vi "Get Connections.vi"(6 "instrument type id":string, 7 "error if pin not found":bool, 8 "error in":errorcluster, 9 "sites":i32[](array[numeric]), 10 "pin or relay names":string[](array[string]), 11 "connection map in":refnum<class "Connection Map.lvclass">) -> (0 "error out":errorcluster, 2 "connections":T1[](array[typedef]), 3 "connection map out":refnum<class "Connection Map.lvclass">)   [LabVIEW 2020, in "MeasurementLink Session Management.lvlib" / "Connection Map.lvclass"]
uses:
  Connection Map.lvclass
  Session Reservation/Connection with Session.ctl
  Session Reservation/Connection.ctl
  Connection Map.lvclass/Connection Map.ctl
  41d5ce38-2fc1-4a99-b6dc-ff10a635fcc4.vi
  MeasurementLink Measurement Server/Helpers/Error Strings Global Internal.vi
  Session Reservation/Session Reservation.lvclass
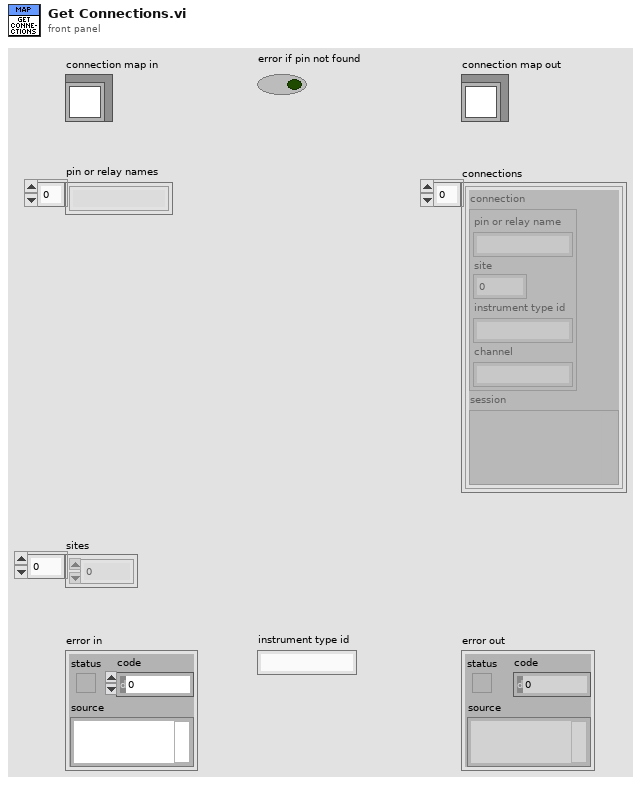
[diagram p1: front panel]
types:
  T1 = typedef "MeasurementLink Session Management.lvlib/Session Reservation.lvclass/Connection with Session.ctl" = cluster{"connection":T2, "session":variant}
  T2 = typedef "MeasurementLink Session Management.lvlib/Session Reservation.lvclass/Connection.ctl" = cluster{"pin or relay name":string, "site":i32, "instrument type id":string, "channel":string}
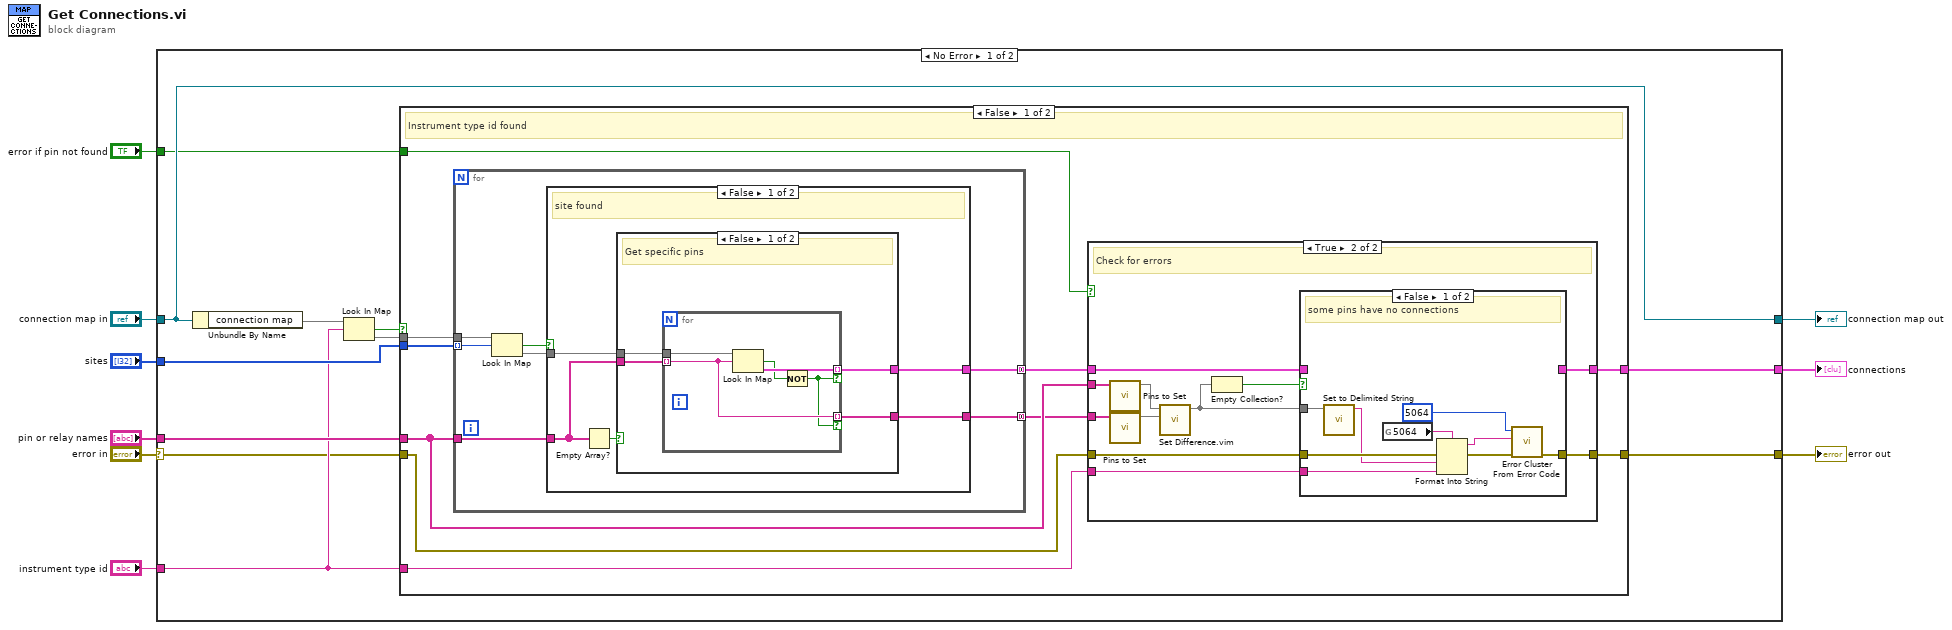
[diagram p0: block diagram]
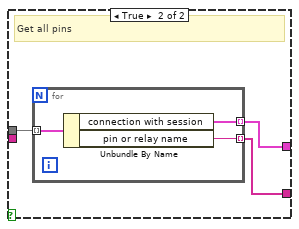
[diagram p2: hidden frame]
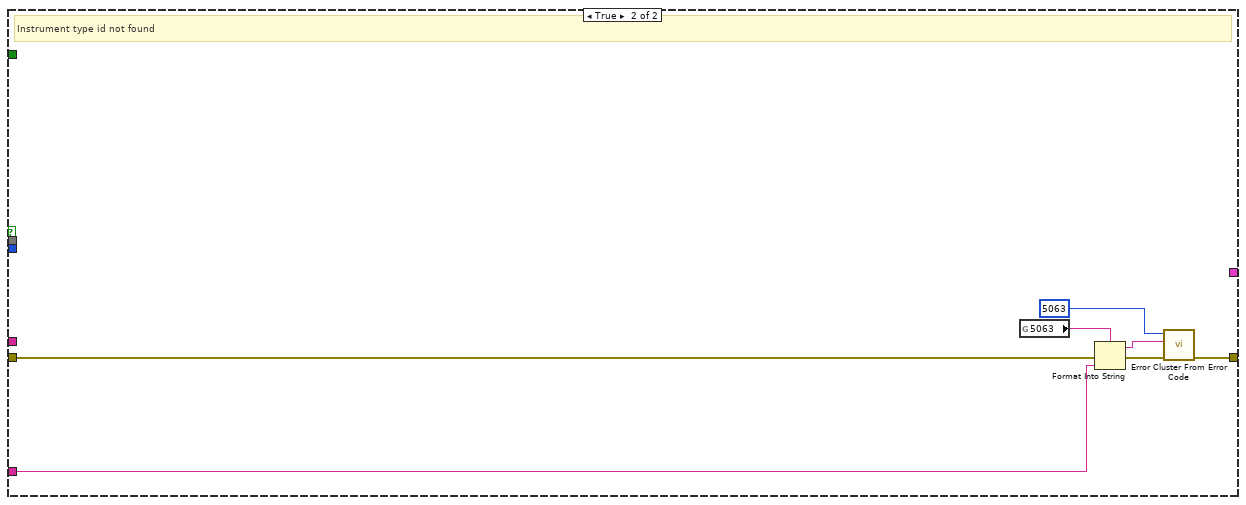
[diagram p6: hidden frame]
diagram:
  n1 = case shown="No Error" "error in" {
    selector: "error in" -> [w11 w90]
    tunnel: [w14 w90] -> w8
    tunnel: [w16 w89] -> w6
    tunnel: "connection map in" -> [w16 w89]
    tunnel: "instrument type id" -> [w13 _]
    tunnel: "sites" -> [w18 _]
    tunnel: "pin or relay names" -> [w17 _]
    tunnel: [w10 _] -> w2
    tunnel: "error if pin not found" -> [w12 _]
    frame No Error {
      n2 = Unbundle By Name(w16) -> ("connection map"=w15:map{string, map{i32, map{string, T1}}})
      n3 = Look In Map(map=w15, key=w13) -> (key not found?=w19:bool, value=w20:map{i32, map{string, T1}})  [unwired: 1 in]
      n4 = case shown="False" w19 {
        tunnel: w20 -> [w30 _]
        tunnel: w18 -> [w29 _]
        tunnel: w17 -> [w22 _]
        tunnel: [w28 _] -> w10
        tunnel: w11 -> [w24 w88]
        tunnel: [w27 w87] -> w14
        tunnel: w13 -> [w25 w86]
        tunnel: w12 -> [w23 _]
        frame False {
          # "Instrument type id found"
          n5 = for {
            tunnel: w30 -> [w37]
            tunnel: w29 -> [w31] mode=indexing
            tunnel: w22 -> [w34]
            tunnel: [w33] -> w26 mode=concatenating
            tunnel: [w32] -> w21 mode=concatenating
            n6 = Look In Map(map=w37, key=w31) -> (key not found?=w36:bool, value=w35:map{string, T1})  [unwired: 1 in]
            n7 = case shown="False" w36 {
              tunnel: w35 -> [w42 _]
              tunnel: w34 -> [w40 _]
              tunnel: [w41 _] -> w33
              tunnel: [w38 _] -> w32
              frame False {
                # "site found"
                n8 = Empty Array?(array=w40) -> (empty?=w39:bool)
                n9 = case shown="False" w39 {
                  tunnel: w42 -> [w46 w54]
                  tunnel: [w44 w53] -> w41
                  tunnel: w40 -> [w45 _]
                  tunnel: [w43 w52] -> w38
                  frame False {
                    # "Get specific pins"
                    n10 = for {
                      tunnel: w46 -> [w51]
                      tunnel: w45 -> [w48] mode=indexing
                      tunnel: [w50] -> w44 mode=indexing if=w47
                      tunnel: [w48] -> w43 mode=indexing if=w47
                      n11 = Look In Map(map=w51, key=w48) -> (key not found?=w49:bool, value=w50:T1)  [unwired: 1 in]
                      n12 = Not(x=w49) -> (.not. x?=w47:bool)
                    }
                  }
                  frame True {
                    # "Get all pins"
                    n13 = for {
                      tunnel: w54 -> [w57] mode=indexing
                      tunnel: [w56] -> w53 mode=indexing
                      tunnel: [w55] -> w52 mode=indexing
                      n14 = Unbundle By Name(w57) -> ("connection with session"=w56:T1, "pin or relay name"=w55:string)
                    }
                  }
                }
              }
              frame True {
                # "site not found"
              }
            }
          }
          n15 = case shown="True" w23 {
            tunnel: [w58 w70] -> w28
            tunnel: [w59 w69] -> w27
            tunnel: w26 -> [w58 w68]
            tunnel: w25 -> [_ w67]
            tunnel: w24 -> [w59 w66]
            tunnel: w22 -> [_ w63]
            tunnel: w21 -> [_ w62]
            frame False {
              # "Don't check for errors"
            }
            frame True {
              # "Check for errors"
              n16 = call "Pins to Set.vi"("pin or relay names array"=w63) -> ("pin or relay name set"=w64:set{string})  [unwired: 10 in]
              n17 = call "Pins to Set.vi"("pin or relay names array"=w62) -> ("pin or relay name set"=w65:set{string})  [unwired: 10 in]
              n18 = call "Set Difference.vim"("set 2"=w65, "set 1"=w64) -> ("difference"=w61:set{string})  [unwired: 9 in]
              n19 = Empty Collection?(1:w61) -> (0:w60:bool)
              n20 = case shown="False" w60 {
                tunnel: w68 -> [_ w81]
                tunnel: [_ w81] -> w70
                tunnel: w66 -> [w75 w80]
                tunnel: [w74 w80] -> w69
                tunnel: w67 -> [w73 _]
                tunnel: w61 -> [w72 _]
                frame False {
                  # "some pins have no connections"
                  n21 = call "Set to Delimited String.vi"("set"=w72) -> ("delimited string"=w71:string)  [unwired: 10 in]
                  n22 = global read "Error Strings Global Internal.vi" "5064"() -> (w79:string)
                  n23 = Format Into String(format string=w79, error in=w75, w71, w73) -> (resulting string=w78:string, error out=w77:errorcluster)  [unwired: 1 in]
                  n24 = call <vilib>:"Error Cluster From Error Code.vi"("error in (no error)"=w77, "error message (\"\")"=w78, "error code (0)"=5064) -> ("error out"=w74:errorcluster)  [unwired: 6 in]
                }
                frame True {
                  # "all pins have connections"
                }
              }
            }
          }
        }
        frame True {
          # "Instrument type id not found"
          n25 = global read "Error Strings Global Internal.vi" "5063"() -> (w83:string)
          n26 = Format Into String(format string=w83, error in=w88, w86) -> (resulting string=w84:string, error out=w85:errorcluster)  [unwired: 1 in]
          n27 = call <vilib>:"Error Cluster From Error Code.vi"("error in (no error)"=w85, "error message (\"\")"=w84, "error code (0)"=5063) -> ("error out"=w87:errorcluster)  [unwired: 6 in]
        }
      }
    }
    frame Error {
    }
  }
  "error out" <- w8
  "connection map out" <- w6
  "connections" <- w2
